vi "CountChassis.vi"(0 "NhRegenGridSim in":refnum<class "NHRGridSim.lvclass">, 11 "error in (no error)":errorcluster) -> (4 "NhRegenGridSim out":refnum<class "NHRGridSim.lvclass">, 6 "Connected?":bool, 8 "Chassis":u32 max=12 step=1, 10 "ChassisTxt":string, 14 "ChassisStatus":T1(ring)=enum."Disabled and Grayed Out", 15 "error out":errorcluster)   [LabVIEW 2018, in "AcPwrPlugins.lvlib" / "NHRGridSim.lvclass"]
uses:
  NHRGridSim.lvclass
  <instrlib>/NH Research 9400 Series/NH Research 9400 Series.lvlib
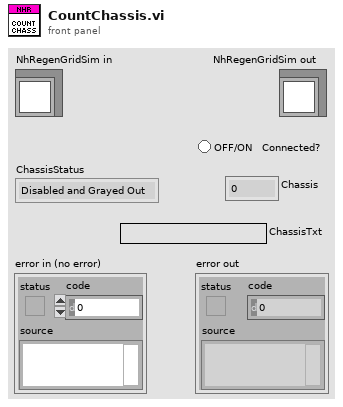
[diagram p1: front panel]
types:
  T1 = enum8{"Enabled", "Disabled", "Disabled and Grayed Out"}
  T2 = typedef "AcPwrPlugins.lvlib/NHRGridSim.lvclass/Device(s)Settings.ctl" = cluster{"MeasName":string, "Instr1":T3, "Instr2":T3, "Instr3":T3, "Handle":string, "Reset":bool, "Mode":T10, "ID Query":bool, "Connected":bool, "Chassis":i32, "VRangeVals1":string[], "ConfList1":string[], "WaveList1":string[], "WaveList2":string[], "WaveList3":string[], "ConfList2":string[], "ConfList3":string[], "VRangeVals3":string[], "VRangeVals2":string[], "CRangeVals1":string[], "CRangeVals3":string[], "CRangeVals2":string[]}
  T3 = typedef "AcPwrPlugins.lvlib/NHRGridSim.lvclass/NHRGrid_InstrumentCluster_Tabs.ctl" = cluster{"Name":string, "Vout (V)":dbl, "VType":string, "Phases":T4, "FreqOut (Hz)":dbl, "Aperture (cycles)":i32, "Configure Instrument":T5, "AC Wave Shape":T6, "Ranges":T7, "Safety Trips":T8, "Slew Rates":T9}
  T4 = typedef "AcPwrPlugins.lvlib/NHRGridSim.lvclass/NHRGrid_Phases_Tabs.ctl" = cluster{"A-Volts (V)":dbl, "B-Volts (V)":dbl, "C-Volts (V)":dbl, "Change at (Deg)":i32, "B-Angle (Deg)":i32, "C-Angle (Deg)":i32}
  T5 = typedef "AcPwrPlugins.lvlib/NHRGridSim.lvclass/NHRGrid_Configure_Tabs.ctl" = u16
  T6 = typedef "AcPwrPlugins.lvlib/NHRGridSim.lvclass/NHRGrid_WaveShape_Tabs.ctl" = u16
  T7 = typedef "AcPwrPlugins.lvlib/NHRGridSim.lvclass/NHRGrid_Ranges_Tabs.ctl" = cluster{"Voltage (V)":u16, "Current (A)":u16}
  T8 = typedef "AcPwrPlugins.lvlib/NHRGridSim.lvclass/NHRGrid_SafetyTrips_Tabs.ctl" = cluster{"Vmax (V)":dbl, "Vmin (V)":dbl, "Vmax Time (s)":dbl, "Vmin Time (s)":dbl, "Imax Source (A)":dbl, "Imax Sink (A)":dbl, "I Src Time (s)":dbl, "I Snk Time (s)":dbl, "Pmax Source (W)":dbl, "Pmax Sink (W)":dbl, "P Src Time (s)":dbl, "P Snk Time (s)":dbl, "Abs Volt Peak":dbl, "Enable Vpk":bool, "Abs Curr Peak":dbl, "Enable Ipk":bool}
  T9 = typedef "AcPwrPlugins.lvlib/NHRGridSim.lvclass/NHRGrid_SlewRates_Tabs.ctl" = cluster{"Voltage (V/s)":dbl, "Current (A/s)":dbl, "Power (W/s)":dbl, "Frequency (Hz/s)":dbl, "Phase Angle (Deg/s)":dbl}
  T10 = typedef "AcPwrPlugins.lvlib/NHRGridSim.lvclass/NHRGrid_Modes.ctl" = u8
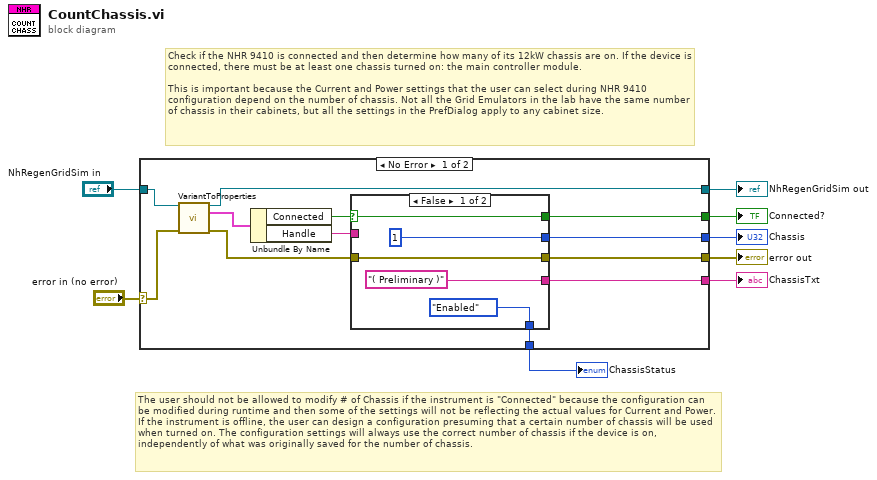
[diagram p0: block diagram]
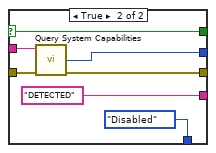
[diagram p2: hidden frame]
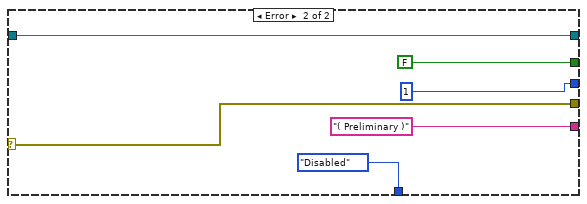
[diagram p3: hidden frame]
diagram:
  # "The user should not be allowed to modify # of Chassis if the instrument is \"Connected\" because the configuration can be modified during runtime and then some of the settings will not be reflecting the actual values for Current and Power. If the instrument is offline, the user can design a configuration presuming that a certain number of chassis will be used when turned on. The configuration settings will always use the correct number of chassis if the device is on, independently of what was originally saved for the number of chassis."
  # "Check if the NHR 9410 is connected and then determine how many of its 12kW chassis are on. If the device is connected, there must be at least one chassis turned on: the main controller module.\n\nThis is important because the Current and Power settings that the user can select during NHR 9410 configuration depend on the number of chassis. Not all the Grid Emulators in the lab have the same number of chassis in their cabinets, but all the settings in the PrefDialog apply to any cabinet size."
  n1 = case shown="No Error" "error in (no error)" {
    selector: "error in (no error)" -> [w19 w38]
    tunnel: [w10 w38] -> w7
    tunnel: "NhRegenGridSim in" -> [w20 w37]
    tunnel: [w17 w37] -> w5
    tunnel: [w14 u32 1 ("Chassis")] -> w4
    tunnel: [w13 "( Preliminary )" ("concatenated string")] -> w3
    tunnel: [w12 FALSE] -> w2
    tunnel: [w9 T1."Disabled" ("Disabled")] -> w1
    frame No Error {
      n2 = call "VariantToProperties.vi"("NHRGridSim in"=w20, "error in (no error)"=w19) -> ("NHRGridSim out"=w17:refnum<class "NHRGridSim.lvclass">, "Device(s)Settings"=w18:T2, "error out"=w11:errorcluster)  [unwired: 8 in, 3 out]
      n3 = Unbundle By Name(w18) -> ("Connected"=w16:bool, "Handle"=w15:string)
      n4 = case shown="False" w16 {
        selector: w16 -> [w23 w29]
        tunnel: w15 -> [_ w32]
        tunnel: [u32 1 ("Chassis") w31] -> w14
        tunnel: ["( Preliminary )" ("concatenated string") "DETECTED" ("concatenated string")] -> w13
        tunnel: [w23 w29] -> w12
        tunnel: w11 -> [w22 w28]
        tunnel: [w22 w27] -> w10
        tunnel: [T1."Enabled" ("Disabled") T1."Disabled" ("Disabled")] -> w9
        frame False {
        }
        frame True {
          n5 = call <instrlib>:"Query System Capabilities.vi"("VISA resource name"=w32, "error in (no error)"=w28) -> ("Chassis"=w31:u32, "error out"=w27:errorcluster)  [unwired: 10 in, 2 out]
        }
      }
    }
    frame Error {
    }
  }
  "error out" <- w7
  "NhRegenGridSim out" <- w5
  "Chassis" <- w4
  "ChassisTxt" <- w3
  "Connected?" <- w2
  "ChassisStatus" <- w1
